vi "msi read test.vi"() -> ()   [LabVIEW 2014]
uses:
  housekeeper/axial_diagnostics/typedefs/7_uwave_MSI_cluster.ctl
panel:
  out "Magnetic field":T1
  out "status 2":u64
  out "error out 2":errorcluster
  out "Waveform Graph 2":sgl[][](graph)
  out "uWave array":T2(array[cluster])
  out "status":u64
  out "error out":errorcluster
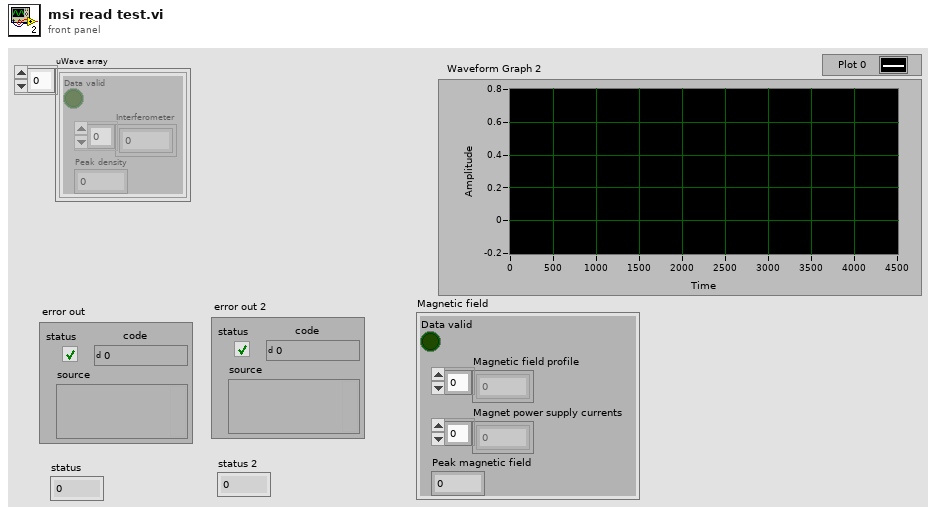
[diagram p1: front panel]
types:
  T1 = cluster{"Data valid":bool, "Magnetic field profile":sgl[], "Magnet power supply currents":sgl[], "Peak magnetic field":sgl}
  T2 = cluster{"Data valid":bool, "Interferometer":sgl[], "Peak density":sgl}[]
  T3 = typedef "7_uwave_MSI_cluster.ctl" = cluster{"Data valid":bool, "Interferometer":sgl[], "Peak density":sgl}[]
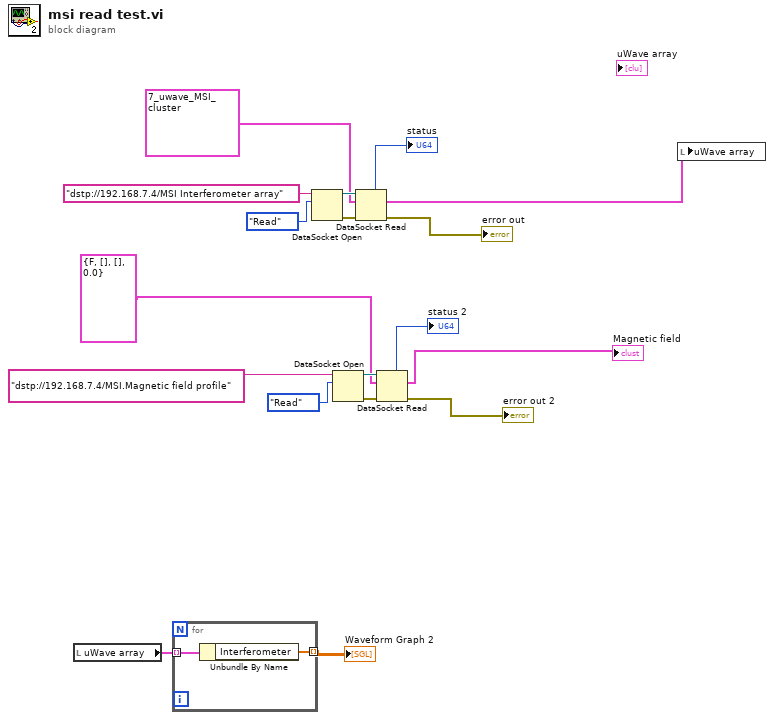
[diagram p0: block diagram]
diagram:
  n1 = local read "uWave array"() -> (w12:T2)
  n2 = for {
    tunnel: w12 -> [w20] mode=indexing
    tunnel: [w19] -> w11 mode=indexing
    n3 = Unbundle By Name(w20) -> ("Interferometer"=w19:sgl[])
  }
  "Waveform Graph 2" <- w11
  n4 = DataSocket Open(10:enum16{"Read"}."Read", 11:"dstp://192.168.7.4/MSI Interferometer array" ("String")) -> (0:w14:errorcluster, 3:w16:refnum<k13>)  [unwired: 2 in]
  n5 = DataSocket Open(10:enum16{"Read"}."Read", 11:"dstp://192.168.7.4/MSI.Magnetic field profile" ("String")) -> (0:w4:errorcluster, 3:w6:refnum<k13>)  [unwired: 2 in]
  n6 = DataSocket Read(8:w14, 10:T3 [{"Data valid"=FALSE, "Interferometer"=array[2048 elements], "Peak density"=0.0}, {"Data valid"=FALSE, "Interferometer"=array[2048 elements], "Peak density"=0.0}, {"Data valid"=FALSE, "Interferometer"=array[2048 elements], "Peak density"=0.0}, {"Data valid"=FALSE, "Interferometer"=array[2048 elements], "Peak density"=0.0}, {"Data valid"=FALSE, "Interferometer"=array[2048 elements], "Peak density"=0.0}, {"Data valid"=FALSE, "Interferometer"=array[2048 elements], "Peak density"=0.0}, {"Data valid"=FALSE, "Interferometer"=array[2048 elements], "Peak density"=0.0}] ("Array"), 11:w16) -> (0:→"error out":errorcluster, 2:w9:T3, 5:→"status":u64)  [unwired: 2 in, 4 out]
  n7 = DataSocket Read(8:w4, 10:T1 {"Data valid"=FALSE, "Magnetic field profile"=[], "Magnet power supply currents"=[], "Peak magnetic field"=0.0} ("Magnetic field"), 11:w6) -> (0:→"error out 2":errorcluster, 2:→"Magnetic field":T1, 5:→"status 2":u64)  [unwired: 2 in, 4 out]
  n8 = local write "uWave array"(w9) -> ()
